vi "err_handle.vi"(2 "retval":i32, 3 "error in":errorcluster) -> (1 "error out":errorcluster)   [LabVIEW 2019, in "msgpack.lvlib"]
doc: "Allocates memory for a msgpack packing object, returned in the pointer p"
uses:
  msgpack.lvlib
panel:
  # "msgpack"
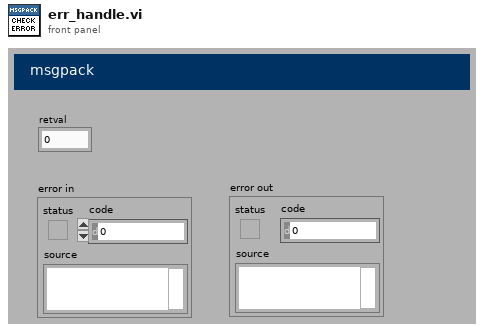
[diagram p1: front panel]
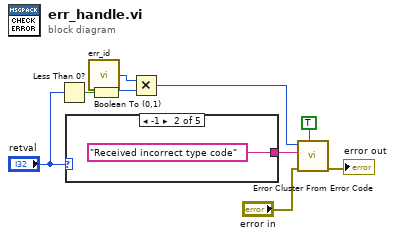
[diagram p0: block diagram]
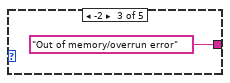
[diagram p3: hidden frame]
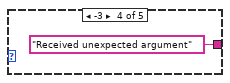
[diagram p4: hidden frame]
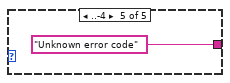
[diagram p5: hidden frame]
diagram:
  n1 = Less Than 0?(x="retval") -> (x < 0?=w4:bool)
  n2 = case shown="-1" "retval" {
    tunnel: [_ "Received incorrect type code" "Out of memory/overrun error" "Received unexpected argument" "Unknown error code"] -> w9
    frame 0.. {
    }
    frame -1 {
    }
    frame -2 {
    }
    frame -3 {
    }
    frame ..-4 {
    }
  }
  n3 = call "err_id.vi"() -> ("error code"=w2:i32)
  n4 = Boolean To (0,1)(Boolean=w4) -> (0, 1=w3:i16)
  n5 = Multiply(x=w2, y=w3) -> (x*y=w1:i32)
  n6 = call <vilib>:"Error Cluster From Error Code.vi"("show call chain? (False)"=TRUE, "error in (no error)"="error in", "error message (\"\")"=w9, "error code (0)"=w1) -> ("error out"=→"error out":errorcluster)  [unwired: 5 in]
